vi "INTERFACE.vi"() -> ()   [LabVIEW 2014]
uses:
  <vilib>/regexp/Match Regular Expression.xnode
  <vilib>/Native 3D Graph/xcontrol/3DPC_SurfacePlot.xctl
panel:
  out "Numeric":dbl
  out "Array YZ":cluster{"y":dbl, "z":dbl}[](array[cluster])
  out "Array XZ":cluster{"x":dbl, "z":dbl}[](array[cluster])
  in  "Menu Tab":enum32{"Page 1", "Page 2"}(tab)
  out "IndIOT":bool
  in  "IOT":bool
  out "IndMnC":bool
  in  "Monitoring and\nControlling":bool
  out "IndCon":bool
  in  "Connection":bool
  out "IndMenu":bool
  in  "Menu":bool
  in  "half":bool
  in  "full":bool
  in  "Main Tab":T1(tab)
  in  "POLMAN":bool
  in  "About":bool
  in  "Exit Program":bool
  in  "Help":bool
  in  "Default":bool
  out "connection status":string
  in  "Disconnect Button":bool
  in  "Connect Button":bool
  in  "Port":string
  in  "IP Address":string
  out "Connection Lamp":bool
  in  "Clear Graph 2":bool
  in  "xyzpict":bool
  in  "Tab Mode":enum32{"Manual", "Automatic"}(tab)
  in  "Spindle Speed Default":bool
  in  "Feeed Rate Default":bool
  in  "Back to Home Button 2":bool
  in  "X+ 2":bool
  in  "X- 2":bool
  in  "Y+ 2":bool
  in  "Y- 2":bool
  in  "Z- 2":bool
  in  "Z+ 2":bool
  in  "Back to Origin":bool
  in  "Set Origin":bool
  in  "Length per Step":string(combo)
  out "Dir":string
  in  "Direction":bool
  in  "set spindle speed":bool
  in  "Spindle Speed Knob":dbl(knob) scale=0.0..4000.0
  out "Spindle Speed":dbl
  in  "Feed Rate Knob":dbl(knob) scale=0.0..1000.0
  out "Feed Rate":dbl
  in  "set feed rate":bool
  in  "Spindle OFF":bool
  in  "Spindle ON":bool
  out "Spindle Lamp":bool
  in  "Stop":bool
  in  "Save":bool
  in  "Clear":bool
  in  "Transfer":bool
  in  "Execute":bool
  in  "Insert":bool
  out "File Name":string
  in  "G-Code List":string
  in  "Address":path
  in  "Tab Graphic":enum32{"3D Graph", "PID Graph", "Speed Graph"}(tab)
  in  "Tab Graph":enum32{"XY Graph", "XZ Graph", "YZ Graph"}(tab)
  out "XY Graph":cluster{"X":dbl, "Y":dbl}[](graph)
  out "XZ Graph":cluster{"X":dbl, "Y":dbl}[](graph)
  out "YZ Graph":cluster{"X":dbl, "Y":dbl}[](graph)
  in  "xy":bool
  in  "xz":bool
  in  "yz":bool
  in  "Save PID Button":bool
  in  "Kd":dbl
  in  "Ki":dbl
  in  "Kp":dbl
  out "Waveform Chart":dbl(graph)
  out "Speed Graph":cluster{"X":dbl, "Y":dbl}[](graph)
  in  "Emergency":bool
  out "Green":bool
  out "Yellow":bool
  out "Red":bool
  out "Status":string
  out "X":dbl
  out "Y":dbl
  out "Z":dbl
  in  "Reset":bool
  in  "Clear Graph":bool
  out "Time":dbl
  out "Speed":cluster{"x":dbl, "y":dbl}[](array[cluster])
  out "Array XY":cluster{"x":dbl, "y":dbl}[](array[cluster])
  out "Data Receive":string
  # "C1 2019"
  # "3 D  E N G R A V I N G"
  # "C1 2019"
  # "Teknik Mekatronika\nPoliteknik Manufaktur Bandung"
  # "CONNECT FIRST!"
  # "CONTROL"
  # "INDICATOR"
  # "URGENCY"
  # "SPINDLE"
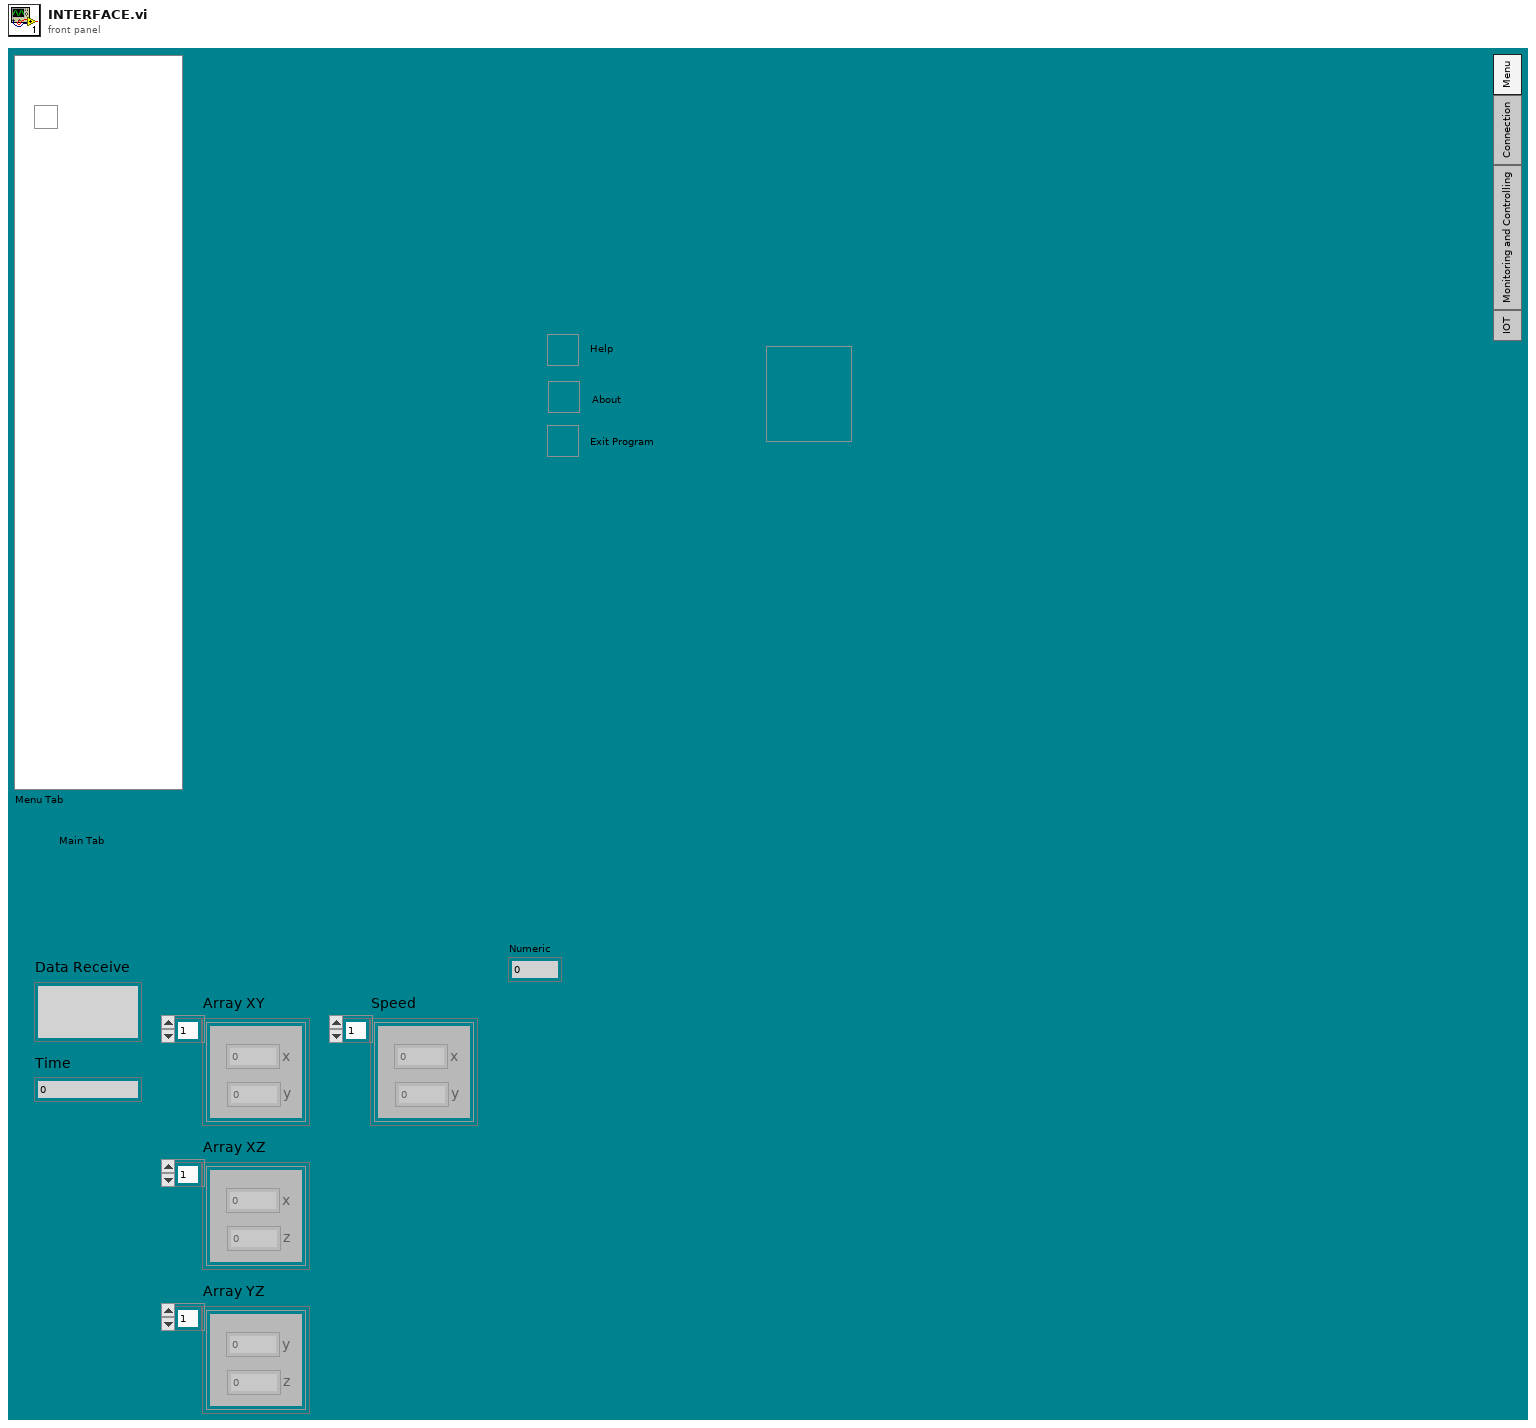
[diagram p1: front panel]
types:
  T1 = enum32{"Menu", "Connection", "Monitoring and Controlling", "IOT"}
  T2 = enum8{"Enabled", "Disabled", "Disabled and Grayed Out"}
  T3 = enum16{"Standard", "Buffered", "CRLF", "Immediate"}
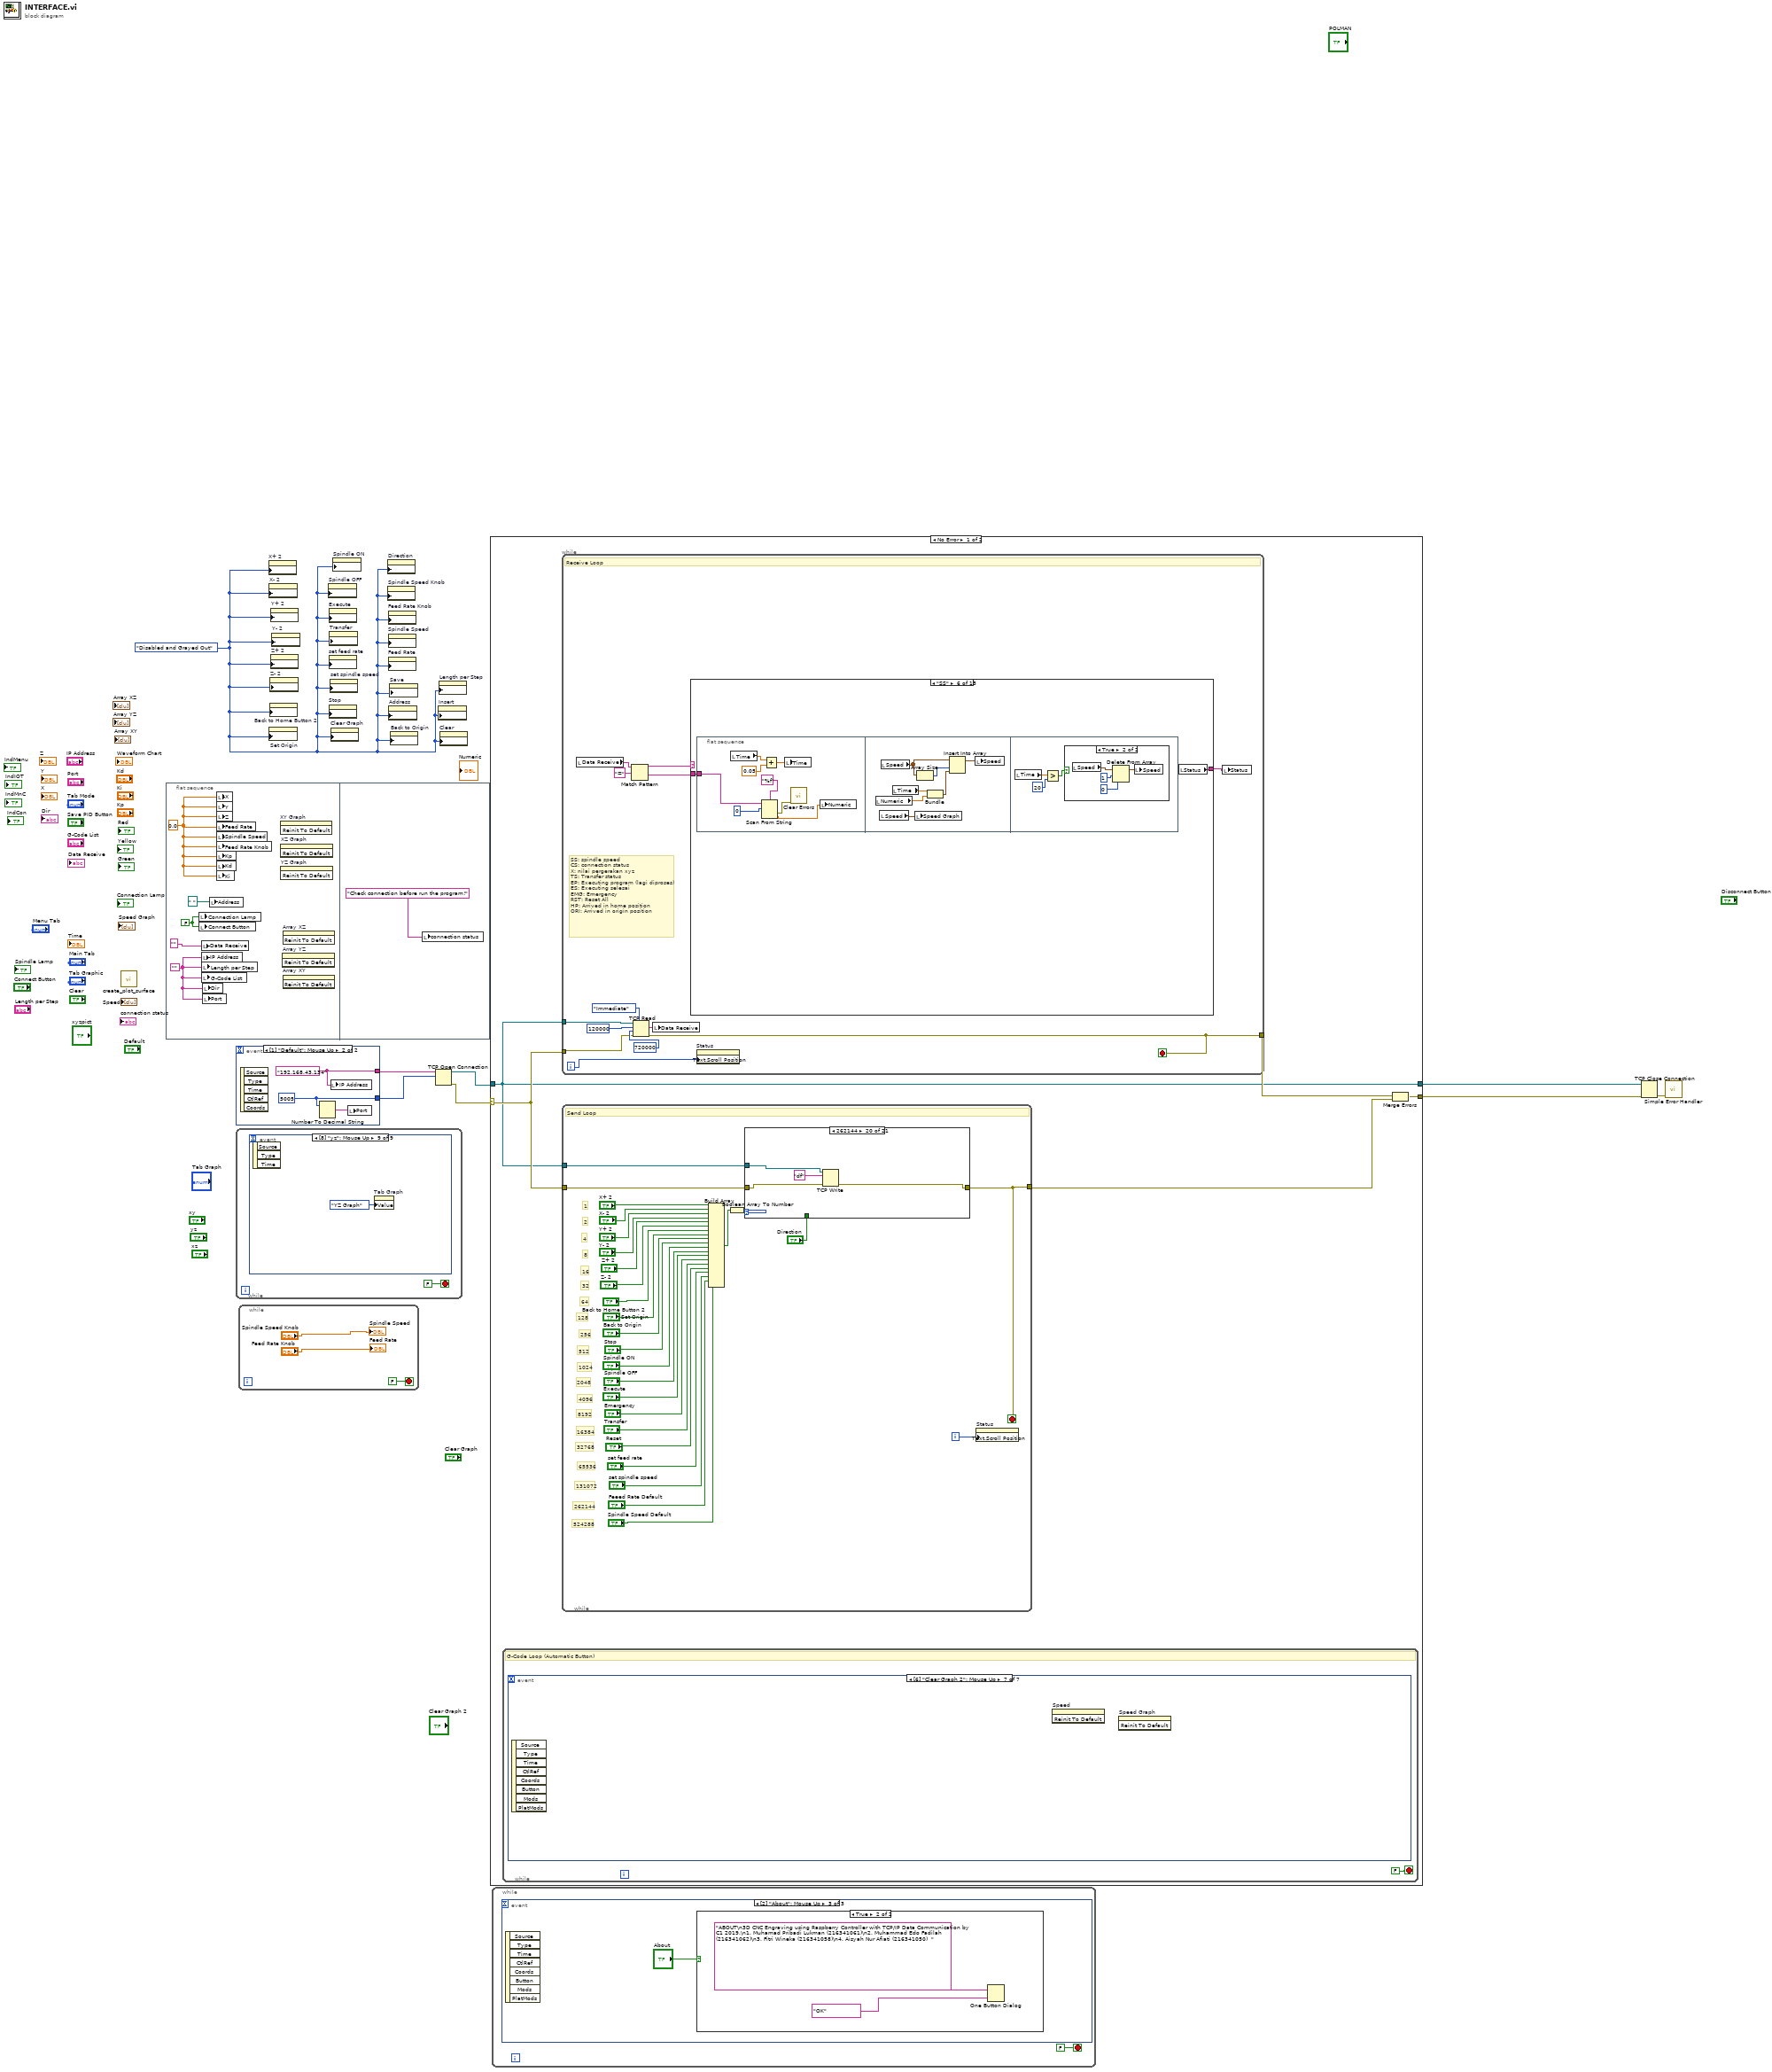
[diagram p0: block diagram]
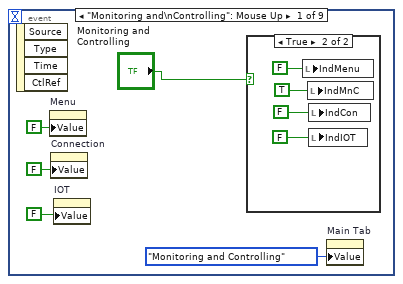
[diagram p2: hidden frame]
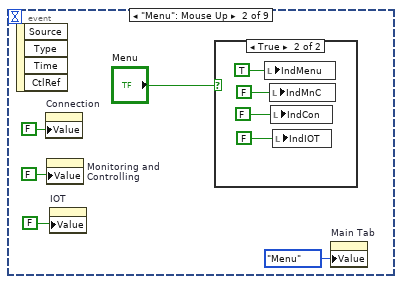
[diagram p4: hidden frame]
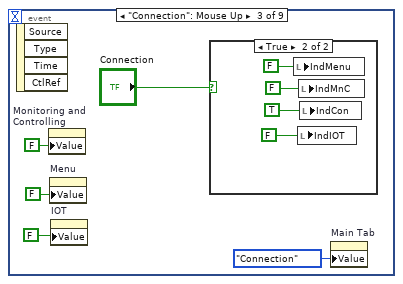
[diagram p6: hidden frame]
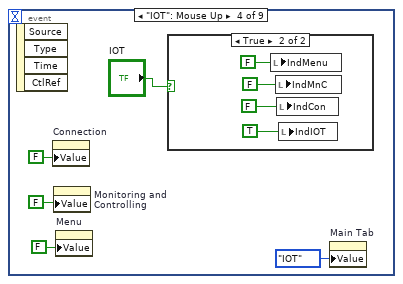
[diagram p8: hidden frame]
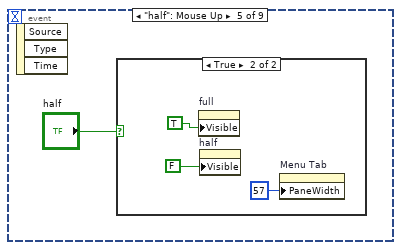
[diagram p10: hidden frame]
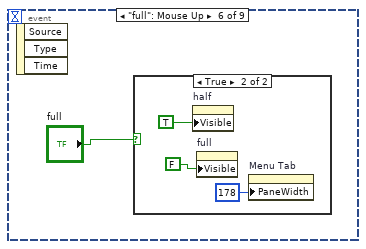
[diagram p12: hidden frame]
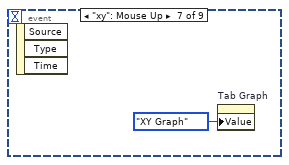
[diagram p14: hidden frame]
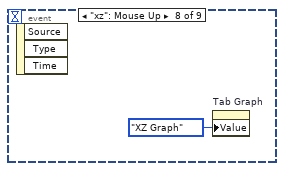
[diagram p15: hidden frame]
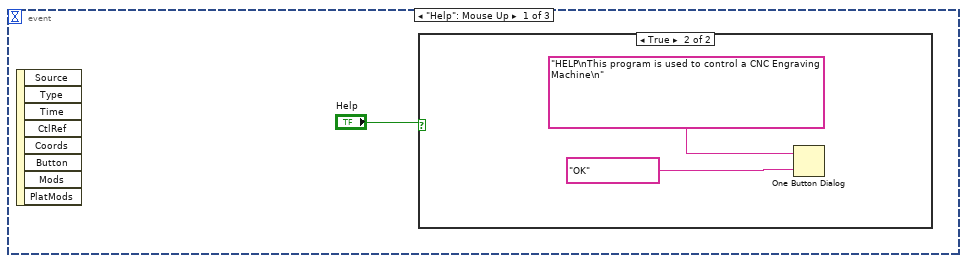
[diagram p16: hidden frame]
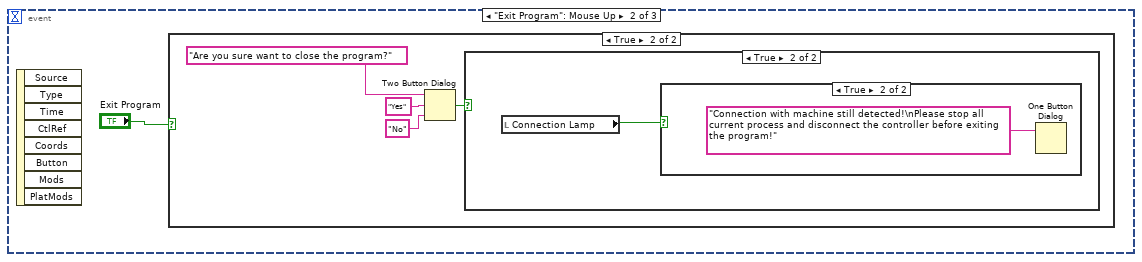
[diagram p18: hidden frame]
diagram:
  w2 = T2."Disabled and Grayed Out" ("Disabled")
  n1 = call <vilib>:"create_plot_surface.vi"() -> ()  [unwired: 5 in, 7 out]
  n2 = flat-sequence {
    frame #0 {
      w11 = FALSE
      w13 = 0.0
      w10 = ""
      n3 = local write "Connection Lamp"(w11) -> ()
      n4 = local write "Connect Button"(w11) -> ()
      n5 = local write "Data Receive"("") -> ()
      n6 = local write "IP Address"(w10) -> ()
      n7 = local write "Length per Step"(w10) -> ()
      n8 = local write "G-Code List"(w10) -> ()
      n9 = local write "Dir"(w10) -> ()
      n10 = local write "Port"(w10) -> ()
      n11 = local write "Address"(path " " ("FILE ADDRESS")) -> ()
      n12 = local write "X"(w13) -> ()
      n13 = local write "Y"(w13) -> ()
      n14 = local write "Z"(w13) -> ()
      n15 = local write "Feed Rate"(w13) -> ()
      n16 = local write "Spindle Speed"(w13) -> ()
      n17 = local write "Feed Rate Knob"(w13) -> ()
      n18 = local write "Kp"(w13) -> ()
      n19 = local write "Kd"(w13) -> ()
      n20 = local write "Ki"(w13) -> ()
      n21 = invoke on="XY Graph" class="XYGraph (strict)" method="Reinit To Default"() -> ()  [unwired: 3 in, 3 out]
      n22 = invoke on="XZ Graph" class="XYGraph (strict)" method="Reinit To Default"() -> ()  [unwired: 3 in, 3 out]
      n23 = invoke on="YZ Graph" class="XYGraph (strict)" method="Reinit To Default"() -> ()  [unwired: 3 in, 3 out]
      n24 = invoke on="Array YZ" class="Arr (strict)" method="Reinit To Default"() -> ()  [unwired: 3 in, 3 out]
      n25 = invoke on="Array XZ" class="Arr (strict)" method="Reinit To Default"() -> ()  [unwired: 3 in, 3 out]
      n26 = invoke on="Array XY" class="Arr (strict)" method="Reinit To Default"() -> ()  [unwired: 3 in, 3 out]
    }
    frame #1 {
      n27 = local write "connection status"("Check connection before run the program!" ("STATUS")) -> ()
    }
  }
  n28 = event shown="[1] \"Default\": Mouse Up" {
    selector: _ -> [_ _]
    dyn-events: _ -> [_ _]
    timeout: _ -> [_ _]
    tunnel: [w17 w20] -> w3
    tunnel: [w15 w18] -> w1
    event "Connect Button": Value Change {
      n29 = event-data() -> ()  [unwired: 1 in, 5 out]
      n30 = local read "Port"() -> (w16:string)
      n31 = local read "IP Address"() -> (w17:string)
      n32 = Decimal String To Number(string=w16) -> (number=w15:i32)  [unwired: 2 in, 1 out]
    }
    event "Default": Mouse Up {
      w20 = "192.168.43.134"
      w18 = 5005
      n33 = event-data() -> ()  [unwired: 1 in, 5 out]
      n34 = Number To Decimal String(number=w18) -> (decimal integer string=w19:string)  [unwired: 1 in]
      n35 = local write "IP Address"(w20) -> ()
      n36 = local write "Port"(w19) -> ()
    }
  }
  n37 = while {
    stop <- FALSE stop-if-true
    n38 = event shown="[8] \"yz\": Mouse Up" {
      selector: _ -> [_ _ _ _ _ _ _ _ _]
      dyn-events: _ -> [_ _ _ _ _ _ _ _ _]
      timeout: _ -> [_ _ _ _ _ _ _ _ _]
      event "Monitoring and\nControlling": Mouse Up {
        n39 = event-data() -> ()  [unwired: 1 in, 4 out]
        n40 = property on="Menu" class="Bool (strict)"("Value"=FALSE ("Menu")) -> ()  [unwired: 2 in, 2 out]
        n41 = property on="Connection" class="Bool (strict)"("Value"=FALSE ("Connection")) -> ()  [unwired: 2 in, 2 out]
        n42 = property on="IOT" class="Bool (strict)"("Value"=FALSE ("Connection")) -> ()  [unwired: 2 in, 2 out]
        n43 = case shown="True" "Monitoring and\nControlling" {
          frame False {
          }
          frame True {
            n44 = local write "IndMenu"(FALSE) -> ()
            n45 = local write "IndMnC"(TRUE) -> ()
            n46 = local write "IndCon"(FALSE) -> ()
            n47 = local write "IndIOT"(FALSE) -> ()
          }
        }
        n48 = property on="Main Tab" class="TabCtl (strict)"("Value"=T1."Monitoring and Controlling" ("Main Tab")) -> ()  [unwired: 2 in, 2 out]
      }
      event "Menu": Mouse Up {
        n49 = event-data() -> ()  [unwired: 1 in, 4 out]
        n50 = property on="Connection" class="Bool (strict)"("Value"=FALSE ("Connection")) -> ()  [unwired: 2 in, 2 out]
        n51 = property on="Monitoring and\nControlling" class="Bool (strict)"("Value"=FALSE ("Connection")) -> ()  [unwired: 2 in, 2 out]
        n52 = property on="IOT" class="Bool (strict)"("Value"=FALSE ("Connection")) -> ()  [unwired: 2 in, 2 out]
        n53 = case shown="True" "Menu" {
          frame False {
          }
          frame True {
            n54 = local write "IndMenu"(TRUE) -> ()
            n55 = local write "IndMnC"(FALSE) -> ()
            n56 = local write "IndCon"(FALSE) -> ()
            n57 = local write "IndIOT"(FALSE) -> ()
          }
        }
        n58 = property on="Main Tab" class="TabCtl (strict)"("Value"=T1."Menu" ("Main Tab")) -> ()  [unwired: 2 in, 2 out]
      }
      event "Connection": Mouse Up {
        n59 = event-data() -> ()  [unwired: 1 in, 4 out]
        n60 = property on="Monitoring and\nControlling" class="Bool (strict)"("Value"=FALSE ("Monitoring and Controlling")) -> ()  [unwired: 2 in, 2 out]
        n61 = property on="Menu" class="Bool (strict)"("Value"=FALSE ("Menu")) -> ()  [unwired: 2 in, 2 out]
        n62 = property on="IOT" class="Bool (strict)"("Value"=FALSE ("Connection")) -> ()  [unwired: 2 in, 2 out]
        n63 = case shown="True" "Connection" {
          frame False {
          }
          frame True {
            n64 = local write "IndMenu"(FALSE) -> ()
            n65 = local write "IndIOT"(FALSE) -> ()
            n66 = local write "IndMnC"(FALSE) -> ()
            n67 = local write "IndCon"(TRUE) -> ()
          }
        }
        n68 = property on="Main Tab" class="TabCtl (strict)"("Value"=T1."Connection" ("Main Tab")) -> ()  [unwired: 2 in, 2 out]
      }
      event "IOT": Mouse Up {
        n69 = event-data() -> ()  [unwired: 1 in, 4 out]
        n70 = property on="Connection" class="Bool (strict)"("Value"=FALSE ("Connection")) -> ()  [unwired: 2 in, 2 out]
        n71 = property on="Monitoring and\nControlling" class="Bool (strict)"("Value"=FALSE ("Connection")) -> ()  [unwired: 2 in, 2 out]
        n72 = property on="Menu" class="Bool (strict)"("Value"=FALSE ("Menu")) -> ()  [unwired: 2 in, 2 out]
        n73 = case shown="True" "IOT" {
          frame False {
          }
          frame True {
            n74 = local write "IndMenu"(FALSE) -> ()
            n75 = local write "IndMnC"(FALSE) -> ()
            n76 = local write "IndCon"(FALSE) -> ()
            n77 = local write "IndIOT"(TRUE) -> ()
          }
        }
        n78 = property on="Main Tab" class="TabCtl (strict)"("Value"=T1."IOT" ("Main Tab")) -> ()  [unwired: 2 in, 2 out]
      }
      event "half": Mouse Up {
        n79 = event-data() -> ()  [unwired: 1 in, 3 out]
        n80 = case shown="True" "half" {
          frame False {
          }
          frame True {
            n81 = property on="full" class="Bool (strict)"("Visible"=TRUE) -> ()  [unwired: 2 in, 2 out]
            n82 = property on="half" class="Bool (strict)"("Visible"=FALSE) -> ()  [unwired: 2 in, 2 out]
            n83 = property on="Menu Tab" class="TabCtl (strict)"("PaneWidth"=u32 57 ("Tab Control Pane Dimension:Height")) -> ()  [unwired: 2 in, 2 out]
          }
        }
      }
      event "full": Mouse Up {
        n84 = event-data() -> ()  [unwired: 1 in, 3 out]
        n85 = case shown="True" "full" {
          frame False {
          }
          frame True {
            n86 = property on="half" class="Bool (strict)"("Visible"=TRUE) -> ()  [unwired: 2 in, 2 out]
            n87 = property on="full" class="Bool (strict)"("Visible"=FALSE) -> ()  [unwired: 2 in, 2 out]
            n88 = property on="Menu Tab" class="TabCtl (strict)"("PaneWidth"=u32 178 ("Tab Control Pane Dimension:Height")) -> ()  [unwired: 2 in, 2 out]
          }
        }
      }
      event "xy": Mouse Up {
        n89 = event-data() -> ()  [unwired: 1 in, 3 out]
        n90 = property on="Tab Graph" class="TabCtl (strict)"("Value"=enum32{"XY Graph", "XZ Graph", "YZ Graph"}."XY Graph" ("Tab Graph")) -> ()  [unwired: 2 in, 2 out]
      }
      event "xz": Mouse Up {
        n91 = event-data() -> ()  [unwired: 1 in, 3 out]
        n92 = property on="Tab Graph" class="TabCtl (strict)"("Value"=enum32{"XY Graph", "XZ Graph", "YZ Graph"}."XZ Graph" ("Tab Graph")) -> ()  [unwired: 2 in, 2 out]
      }
      event "yz": Mouse Up {
        n93 = event-data() -> ()  [unwired: 1 in, 3 out]
        n94 = property on="Tab Graph" class="TabCtl (strict)"("Value"=enum32{"XY Graph", "XZ Graph", "YZ Graph"}."YZ Graph" ("Tab Graph")) -> ()  [unwired: 2 in, 2 out]
      }
    }
  }
  n95 = while {
    stop <- FALSE stop-if-true
    "Feed Rate" <- "Feed Rate Knob"
    "Spindle Speed" <- "Spindle Speed Knob"
  }
  n96 = property on="X+ 2" class="Bool"("DisabledEnum"=w2) -> ()  [unwired: 2 in, 2 out]
  n97 = property on="X- 2" class="Bool"("DisabledEnum"=w2) -> ()  [unwired: 2 in, 2 out]
  n98 = property on="Set Origin" class="Bool"("DisabledEnum"=w2) -> ()  [unwired: 2 in, 2 out]
  n99 = property on="Back to Home Button 2" class="Bool"("DisabledEnum"=w2) -> ()  [unwired: 2 in, 2 out]
  n100 = property on="Z- 2" class="Bool"("DisabledEnum"=w2) -> ()  [unwired: 2 in, 2 out]
  n101 = property on="Y+ 2" class="Bool"("DisabledEnum"=w2) -> ()  [unwired: 2 in, 2 out]
  n102 = property on="Z+ 2" class="Bool"("DisabledEnum"=w2) -> ()  [unwired: 2 in, 2 out]
  n103 = property on="Y- 2" class="Bool"("DisabledEnum"=w2) -> ()  [unwired: 2 in, 2 out]
  n104 = property on="Spindle OFF" class="Bool"("DisabledEnum"=w2) -> ()  [unwired: 2 in, 2 out]
  n105 = property on="Execute" class="Bool"("DisabledEnum"=w2) -> ()  [unwired: 2 in, 2 out]
  n106 = property on="set feed rate" class="Bool"("DisabledEnum"=w2) -> ()  [unwired: 2 in, 2 out]
  n107 = property on="Stop" class="Bool"("DisabledEnum"=w2) -> ()  [unwired: 2 in, 2 out]
  n108 = property on="Transfer" class="Bool"("DisabledEnum"=w2) -> ()  [unwired: 2 in, 2 out]
  n109 = property on="set spindle speed" class="Bool"("DisabledEnum"=w2) -> ()  [unwired: 2 in, 2 out]
  n110 = property on="Clear Graph" class="Bool (strict)"("DisabledEnum"=w2) -> ()  [unwired: 2 in, 2 out]
  n111 = property on="Spindle ON" class="Bool"("DisabledEnum"=w2) -> ()  [unwired: 2 in, 2 out]
  n112 = property on="Direction" class="Bool (strict)"("DisabledEnum"=w2) -> ()  [unwired: 2 in, 2 out]
  n113 = property on="Spindle Speed Knob" class="Knob (strict)"("DisabledEnum"=w2) -> ()  [unwired: 2 in, 2 out]
  n114 = property on="Feed Rate Knob" class="Knob (strict)"("DisabledEnum"=w2) -> ()  [unwired: 2 in, 2 out]
  n115 = property on="Spindle Speed" class="DigNum (strict)"("DisabledEnum"=w2) -> ()  [unwired: 2 in, 2 out]
  n116 = property on="Feed Rate" class="DigNum (strict)"("DisabledEnum"=w2) -> ()  [unwired: 2 in, 2 out]
  n117 = property on="Address" class="Path"("DisabledEnum"=w2) -> ()  [unwired: 2 in, 2 out]
  n118 = property on="Save" class="Bool (strict)"("DisabledEnum"=w2) -> ()  [unwired: 2 in, 2 out]
  n119 = property on="Back to Origin" class="Bool"("DisabledEnum"=w2) -> ()  [unwired: 2 in, 2 out]
  n120 = TCP Open Connection(address=w3, remote port or service name=w1) -> (connection ID=w7:refnum<k5>, error out=w8:errorcluster)  [unwired: 3 in]
  n121 = property on="Insert" class="Bool (strict)"("DisabledEnum"=w2) -> ()  [unwired: 2 in, 2 out]
  n122 = property on="Length per Step" class="CmbBox"("DisabledEnum"=w2) -> ()  [unwired: 2 in, 2 out]
  n123 = property on="Clear" class="Bool (strict)"("DisabledEnum"=w2) -> ()  [unwired: 2 in, 2 out]
  n124 = case shown="No Error" w8 {
    selector: w8 -> [w75 w1079]
    tunnel: w7 -> [w74 w1080]
    tunnel: [w72 w1079] -> w6
    tunnel: [w74 w1080] -> w4
    frame No Error {
      n125 = while {
        stop <- FALSE stop-if-true
        # "G-Code Loop (Automatic Button)"
        n126 = event shown="[6] \"Clear Graph 2\": Mouse Up" {
          selector: _ -> [_ _ _ _ _ _ _]
          dyn-events: _ -> [_ _ _ _ _ _ _]
          timeout: _ -> [_ _ _ _ _ _ _]
          event "Insert": Mouse Up {
            n127 = event-data() -> ()  [unwired: 1 in, 8 out]
            n128 = case shown="True" "Insert" {
              frame False {
              }
              frame True {
                w84 = "Open G-Code Manually"  # prompt (open existing file)
                n129 = Read from Text File(prompt (Open existing file)=w84) -> (refnum out=w80:refnum<file>, text=w82:string, cancelled=w81:bool, error out=w83:errorcluster)  [unwired: 3 in]
                n130 = call <vilib>:"Clear Errors.vi"("error in (no error)"=w83) -> ()  [unwired: 5 in, 2 out]
                n131 = case shown="False" w81 {
                  tunnel: w82 -> [_ w90]
                  tunnel: ["Cancelled" w89] -> w79
                  tunnel: w80 -> [_ w87]
                  frame True {
                  }
                  frame False {
                    n132 = Refnum to Path(1:w87) -> (0:w95:path)
                    n133 = Strip Path(path=w95) -> (name=w91:string)  [unwired: 1 out]
                    n134 = xnode ("Match Regular Expression")("input string"=w91, "regular expression"=".nc", "ignore case? (F)"=TRUE) -> ("whole match"=w94:string)  [unwired: 3 in, 4 out]
                    n135 = Printable?(1:w94) -> (0:w88:bool)
                    n136 = case shown="False" w88 {
                      tunnel: ["File is not compatible." "File opened"] -> w89
                      tunnel: w91 -> [_ _]
                      tunnel: w90 -> [_ w100]
                      tunnel: ["" w100] -> w86
                      frame False {
                        n137 = One Button Dialog(message="The file you are trying to open is not compatible with this program.", button name ("OK")="OK") -> ()  [unwired: 1 out]
                      }
                      frame True {
                      }
                    }
                    n138 = local write "G-Code List"(w86) -> ()
                  }
                }
                n139 = local write "Status"(w79) -> ()
              }
            }
          }
          event "Address": Value Change {
            n140 = event-data() -> ()  [unwired: 1 in, 6 out]
            n141 = flat-sequence {
              tunnel: [w224] -> w219
              tunnel: [w223] -> w218
              tunnel: [w222] -> w217
              tunnel: [w221] -> w216
              tunnel: w219 -> [w493]
              tunnel: w218 -> [w494]
              tunnel: w217 -> [w495]
              tunnel: w216 -> [w496]
              frame #0 {
                n142 = Strip Path(path="Address") -> (stripped path=w236:path, name=w235:string)
                n143 = xnode "Match Regular Expression"("input string"=w235, "regular expression"=".dxf", "ignore case? (F)"=FALSE) -> ("before match"=w233:string, "whole match"=w232:string)  [unwired: 3 in, 3 out]
                n144 = Printable?(1:w232) -> (0:w225:bool)
                n145 = case shown="False" w225 {
                  tunnel: w236 -> [w372 w488]
                  tunnel: w235 -> [w369 w489]
                  tunnel: w233 -> [_ w490]
                  tunnel: "Address" -> [w365 w487]
                  tunnel: [w366 FALSE] -> w226
                  tunnel: [w367 w490] -> w227
                  tunnel: [w369 w489] -> w229
                  tunnel: [w372 w488] -> w228
                  tunnel: [w365 w487] -> w230
                  frame False {
                    n146 = xnode "Match Regular Expression"("input string"=w369, "regular expression"=".stl", "ignore case? (F)"=TRUE) -> ("before match"=w367:string, "whole match"=w368:string)  [unwired: 3 in, 3 out]
                    n147 = Printable?(1:w368) -> (0:w366:bool)
                  }
                  frame True {
                  }
                }
                n148 = Or(x=w226, y=w225) -> (x .or. y?=w221:bool)
                n149 = case shown="False" w221 {
                  tunnel: w230 -> [_ w250]
                  tunnel: w229 -> [_ w243]
                  tunnel: w228 -> [_ w242]
                  tunnel: w227 -> [_ w241]
                  tunnel: [w238 w243] -> w223
                  tunnel: [w237 w242] -> w224
                  tunnel: [w238 w241] -> w222
                  frame False {
                    w238 = ""
                    w237 = path ""
                    n150 = One Button Dialog(message="The file you are trying to open is not compatible with this program.", button name ("OK")="OK") -> ()  [unwired: 1 out]
                    n151 = local write "Address"(w237) -> ()
                  }
                  frame True {
                    n152 = Path To String(path=w250) -> (string=w248:string)
                    n153 = Concatenate Strings("cmd /c\"", w248, "\"") -> (w246:string)
                    n154 = call <vilib>:"System Exec.vi"("run minimized? (F)"=FALSE, "wait until completion? (T)"=TRUE, "command line"=w246) -> ()  [unwired: 5 in, 4 out]
                  }
                }
              }
              frame #1 {
                n155 = case shown="True" w496 {
                  tunnel: w495 -> [_ w506]
                  tunnel: w494 -> [_ w498]
                  tunnel: w493 -> [_ w503]
                  tunnel: ["File is not compatible." w499] -> w492
                  frame False {
                  }
                  frame True {
                    n156 = Concatenate Strings(w506, ".nc") -> (w504:string)
                    n157 = Build Path(base path=w503, name or relative path=w504) -> (appended path=w502:path)
                    n158 = Read from Text File(file (use dialog)=w502) -> (text=w500:string, error out=w501:errorcluster)  [unwired: 3 in, 2 out]
                    n159 = case shown="Error" w501 {
                      tunnel: w500 -> [_ _]
                      tunnel: ["File opened" w508] -> w499
                      frame No Error {
                      }
                      frame Error {
                        n160 = Two Button Dialog(message="Your G-Code file may has different name or location as your 3D file. Do you want to browse it manually?", 1:"No", 2:"Yes") -> (T button?=w509:bool)
                        n161 = case shown="True" w509 {
                          tunnel: ["Cancelled" w514] -> w508
                          frame False {
                          }
                          frame True {
                            n162 = Read from Text File(prompt (Open existing file)="Open G-Code manually") -> (refnum out=w515:refnum<file>, text=w516:string, cancelled=w517:bool, error out=w518:errorcluster)  [unwired: 3 in]
                            n163 = call <vilib>:"Clear Errors.vi"("error in (no error)"=w518) -> ()  [unwired: 5 in, 2 out]
                            n164 = case shown="False" w517 {
                              tunnel: w516 -> [w525 _]
                              tunnel: w515 -> [w531 _]
                              tunnel: [w522 "Cancelled"] -> w514
                              frame False {
                                n165 = Refnum to Path(1:w531) -> (0:w524:path)
                                n166 = Strip Path(path=w524) -> (name=w526:string)  [unwired: 1 out]
                                n167 = xnode "Match Regular Expression"("input string"=w526, "regular expression"=".nc", "ignore case? (F)"=TRUE) -> ("whole match"=w528:string)  [unwired: 3 in, 4 out]
                                n168 = Printable?(1:w528) -> (0:w527:bool)
                                n169 = case shown="False" w527 {
                                tunnel: w526 -> [_ w539]
                                tunnel: w525 -> [_ w538]
                                tunnel: w524 -> [_ w540]
                                tunnel: [path "" w540] -> w521
                                tunnel: [w534 w539] -> w523
                                tunnel: [w534 w538] -> w520
                                tunnel: ["File is not compatible" "File opened"] -> w522
                                frame False {
                                w534 = ""
                                n170 = One Button Dialog(message="The file you are trying to open has different file format.", button name ("OK")="OK") -> ()  [unwired: 1 out]
                                }
                                frame True {
                                }
                                }
                                n171 = local write "File Name"(w523) -> ()
                                n172 = local write "G-Code List"(w520) -> ()
                                n173 = local write "Address"(w521) -> ()
                              }
                              frame True {
                              }
                            }
                          }
                        }
                      }
                    }
                    "File Name" <- w498
                  }
                }
                "Status" <- w492
              }
            }
          }
          event "Save": Value Change {
            n174 = event-data() -> ()  [unwired: 1 in, 6 out]
            n175 = case shown="True" "Save" {
              frame False {
              }
              frame True {
                n176 = property on="G-Code List" class="Str"() -> ("Text.Text"=w657:string)  [unwired: 2 in, 2 out]
                n177 = Write to Text File(prompt (Choose or enter file path)="Save", text=w657) -> (cancelled=w660:bool, error out=w659:errorcluster)  [unwired: 2 in, 1 out]
                n178 = case shown="True" w660 {
                  tunnel: ["G-Code file is saved" "Cancelled saving"] -> w658
                  frame False {
                  }
                  frame True {
                  }
                }
                n179 = call <vilib>:"Clear Errors.vi"("error in (no error)"=w659) -> ()  [unwired: 5 in, 2 out]
                n180 = local write "Status"(w658) -> ()
              }
            }
          }
          event "Reset": Mouse Up {
            w664 = ""
            n181 = event-data() -> ()  [unwired: 1 in, 8 out]
            n182 = local write "File Name"(w664) -> ()
            n183 = local write "Address"(path "") -> ()
            n184 = local write "G-Code List"(w664) -> ()
            n185 = local write "Status"(w664) -> ()
          }
          event "Clear": Mouse Up {
            w667 = ""
            n186 = event-data() -> ()  [unwired: 1 in, 8 out]
            n187 = local write "Length per Step"(w667) -> ()
            n188 = local write "G-Code List"(w667) -> ()
            n189 = local write "File Name"(w667) -> ()
            n190 = local write "Status"(w667) -> ()
            n191 = local write "Address"(path "") -> ()
          }
          event "Clear Graph": Mouse Up {
            w668 = 0.0
            n192 = event-data() -> ()  [unwired: 1 in, 8 out]
            n193 = invoke on="XY Graph" class="XYGraph (strict)" method="Reinit To Default"() -> ()  [unwired: 3 in, 3 out]
            n194 = invoke on="XZ Graph" class="XYGraph (strict)" method="Reinit To Default"() -> ()  [unwired: 3 in, 3 out]
            n195 = invoke on="YZ Graph" class="XYGraph (strict)" method="Reinit To Default"() -> ()  [unwired: 3 in, 3 out]
            n196 = invoke on="Array YZ" class="Arr (strict)" method="Reinit To Default"() -> ()  [unwired: 3 in, 3 out]
            n197 = invoke on="Array XZ" class="Arr (strict)" method="Reinit To Default"() -> ()  [unwired: 3 in, 3 out]
            n198 = invoke on="Array XY" class="Arr (strict)" method="Reinit To Default"() -> ()  [unwired: 3 in, 3 out]
            n199 = local write "X"(w668) -> ()
            n200 = local write "Y"(w668) -> ()
            n201 = local write "Z"(w668) -> ()
          }
          event "Clear Graph 2": Mouse Up {
            n202 = event-data() -> ()  [unwired: 1 in, 8 out]
            n203 = invoke on="Speed" class="Arr (strict)" method="Reinit To Default"() -> ()  [unwired: 3 in, 3 out]
            n204 = invoke on="Speed Graph" class="XYGraph (strict)" method="Reinit To Default"() -> ()  [unwired: 3 in, 3 out]
          }
        }
      }
      n205 = while {
        tunnel: w74 -> [w901]
        tunnel: w75 -> [w900]
        tunnel: [w899] -> w76
        i -> [w898]
        stop <- w899 stop-if-true
        # "SS: spindle speed\nCS: connection status\nX: nilai pergerakan xyz\nTS: Transfer status\nEP: Executing program (lagi diproses)\nES: Executing selesai\nEMG: Emergency\nRST: Reset All\nHP: Arrived in home position\nORI: Arrived in origin position"
        # "Receive Loop"
        n206 = local read "Data Receive"() -> (w895:string)
        n207 = Match Pattern(string=w895, regular expression="=") -> (before substring=w897:string, after substring=w893:string)  [unwired: 1 in, 2 out]
        n208 = TCP Read(connection ID=w901, bytes to read=120000, error in (no error)=w900, 7:T3."Immediate" ("mode (standard)"), 9:720000) -> (data out=w902:string, error out=w899:errorcluster)  [unwired: 1 out]
        n209 = local write "Data Receive"(w902) -> ()
        n210 = case shown="\"SS\"" w897 {
          tunnel: w893 -> [_ w907 _ _ _ w976 _ _ _ _ _ _ _]
          tunnel: [w906 w908 w943 w956 w966 w977 "" w1008 w1026 w1036 w1046 w1057 w1067] -> w894
          frame "0", Default {
            n211 = local read "Status"() -> (w906:string)
          }
          frame "X" {
            n212 = flat-sequence {
              tunnel: w907 -> [w909]
              frame #0 {
                n213 = Scan From String "Scan From String"(format string="%fY%fZ%f", input string=w909, initial scan location=u32 0) -> (error out=w914:errorcluster, output 1=w912:dbl, output 2=w911:dbl, output 3=w910:dbl)  [unwired: 4 in, 2 out]
                n214 = call <vilib>:"Clear Errors.vi"("error in (no error)"=w914) -> ()  [unwired: 5 in, 2 out]
                n215 = local write "X"(w912) -> ()
                n216 = local write "Y"(w911) -> ()
                n217 = local write "Z"(w910) -> ()
              }
              frame #1 {
                n218 = local read "Array XY"() -> (w941:cluster{"x":dbl, "y":dbl}[])
                n219 = local read "X"() -> (w925:dbl)
                n220 = local read "Y"() -> (w926:dbl)
                n221 = local read "Array XZ"() -> (w936:cluster{"x":dbl, "z":dbl}[])
                n222 = local read "X"() -> (w923:dbl)
                n223 = local read "Z"() -> (w924:dbl)
                n224 = local read "Array YZ"() -> (w935:cluster{"y":dbl, "z":dbl}[])
                n225 = local read "Y"() -> (w922:dbl)
                n226 = local read "Z"() -> (w933:dbl)
                n227 = local read "Array XY"() -> (w918:cluster{"x":dbl, "y":dbl}[])
                n228 = local read "Array XZ"() -> (w917:cluster{"x":dbl, "z":dbl}[])
                n229 = local read "Array YZ"() -> (w916:cluster{"y":dbl, "z":dbl}[])
                n230 = Array Size(array=w941) -> (size(s)=w939:i32)
                n231 = Bundle("X"=w925, "Y"=w926) -> (w940:cluster{"X":dbl, "Y":dbl})  [unwired: 1 in]
                n232 = Bundle("Y"=w926, "X"=w925) -> (w921:cluster{"Y":dbl, "X":dbl})  [unwired: 1 in]
                n233 = Array Size(array=w936) -> (size(s)=w938:i32)
                n234 = Bundle("X"=w923, "Z"=w924) -> (w937:cluster{"X":dbl, "Z":dbl})  [unwired: 1 in]
                n235 = Bundle("Z"=w924, "X"=w923) -> (w920:cluster{"Z":dbl, "X":dbl})  [unwired: 1 in]
                n236 = Array Size(array=w935) -> (size(s)=w932:i32)
                n237 = Bundle("Y"=w922, "Z"=w933) -> (w934:cluster{"Y":dbl, "Z":dbl})  [unwired: 1 in]
                n238 = Bundle("Y"=w922, "Y"=w922) -> (w919:cluster{"Y":dbl, "Y":dbl})  [unwired: 1 in]
                n239 = Insert Into Array(array=w941, index=w939, new element=w940) -> (w942:cluster{"x":dbl, "y":dbl}[])
                n240 = Insert Into Array(array=w936, index=w938, new element=w937) -> (w931:cluster{"x":dbl, "z":dbl}[])
                n241 = Build Array (concatenate)(w921, w918) -> (→"XY Graph":cluster{"x":dbl, "y":dbl}[])
                n242 = Build Array (concatenate)(w920, w917) -> (→"XZ Graph":cluster{"x":dbl, "z":dbl}[])
                n243 = Insert Into Array(array=w935, index=w932, new element=w934) -> (w930:cluster{"y":dbl, "z":dbl}[])
                n244 = Build Array (concatenate)(w919, w916) -> (→"YZ Graph":cluster{"y":dbl, "z":dbl}[])
                n245 = local write "Array XY"(w942) -> ()
                n246 = local write "Array YZ"(w930) -> ()
                n247 = local write "Array XZ"(w931) -> ()
              }
            }
            n248 = local read "Status"() -> (w908:string)
          }
          frame "TS" {
            n249 = local read "Status"() -> (w947:string)
            n250 = Equal?(x=w947, y="") -> (x = y?=w945:bool)
            n251 = case shown="False" w945 {
              tunnel: "G-Code is transferred successfully.\nYou may execute the program" -> [w948 w952]
              tunnel: [w949 w952] -> w943
              frame False {
                n252 = local read "Status"() -> (w950:string)
                n253 = Concatenate Strings(w950, "\r", w948) -> (w949:string)
              }
              frame True {
              }
            }
          }
          frame "EP" {
            n254 = local read "Status"() -> (w957:string)
            n255 = local write "Yellow"(FALSE) -> ()
            n256 = local write "Green"(TRUE) -> ()
            n257 = local write "Red"(FALSE) -> ()
            n258 = Equal?(x=w957, y="") -> (x = y?=w959:bool)
            n259 = case shown="False" w959 {
              tunnel: "Executing the program..." -> [w962 w965]
              tunnel: [w961 w965] -> w956
              frame False {
                n260 = local read "Status"() -> (w963:string)
                n261 = Concatenate Strings(w963, "\r", w962) -> (w961:string)
              }
              frame True {
              }
            }
          }
          frame "ES" {
            n262 = local read "Status"() -> (w968:string)
            n263 = Equal?(x=w968, y="") -> (x = y?=w967:bool)
            n264 = case shown="False" w967 {
              tunnel: "The program has been fully executed" -> [w972 w975]
              tunnel: [w971 w975] -> w966
              frame False {
                n265 = local read "Status"() -> (w974:string)
                n266 = Concatenate Strings(w974, "\r", w972) -> (w971:string)
              }
              frame True {
              }
            }
          }
          frame "SS" {
            n267 = flat-sequence {
              tunnel: w976 -> [w982]
              frame #0 {
                n268 = local read "Time"() -> (w985:dbl)
                n269 = Scan From String "Scan From String"(format string="%f", input string=w982, initial scan location=u32 0) -> (error out=w981:errorcluster, output 1=w978:dbl)  [unwired: 2 in, 2 out]
                n270 = Add(x=w985, y=0.05) -> (x+y=w983:dbl)
                n271 = local write "Time"(w983) -> ()
                n272 = call <vilib>:"Clear Errors.vi"("error in (no error)"=w981) -> ()  [unwired: 5 in, 2 out]
                n273 = local write "Numeric"(w978) -> ()
              }
              frame #1 {
                n274 = local read "Numeric"() -> (w989:dbl)
                n275 = local read "Speed"() -> (w986:cluster{"x":dbl, "y":dbl}[])
                n276 = local read "Speed"() -> (w991:cluster{"x":dbl, "y":dbl}[])
                n277 = local read "Time"() -> (w988:dbl)
                n278 = local write "Speed Graph"(w986) -> ()
                n279 = Array Size(array=w991) -> (size(s)=w992:i32)
                n280 = Bundle("Time"=w988, "Numeric"=w989) -> (w987:cluster{"Time":dbl, "Numeric":dbl})  [unwired: 1 in]
                n281 = Insert Into Array(array=w991, index=w992, new element=w987) -> (w990:cluster{"x":dbl, "y":dbl}[])
                n282 = local write "Speed"(w990) -> ()
              }
              frame #2 {
                n283 = local read "Time"() -> (w995:dbl)
                n284 = Greater?(x=w995, y=20) -> (0:w994:bool)
                n285 = case shown="True" w994 {
                  frame False {
                  }
                  frame True {
                    n286 = local read "Speed"() -> (w997:cluster{"x":dbl, "y":dbl}[])
                    n287 = Delete From Array(array=w997, length=1, index=0) -> (array with subset deleted=w996:cluster{"x":dbl, "y":dbl}[])  [unwired: 1 out]
                    n288 = local write "Speed"(w996) -> ()
                  }
                }
              }
            }
            n289 = local read "Status"() -> (w977:string)
          }
          frame "CS" {
            w1000 = T2."Enabled" ("Disabled")
            n290 = local write "Connection Lamp"(TRUE) -> ()
            n291 = local write "connection status"("You have successfully connected controller") -> ()
            n292 = property on="X+ 2" class="Bool"("DisabledEnum"=w1000) -> ()  [unwired: 2 in, 2 out]
            n293 = property on="X- 2" class="Bool"("DisabledEnum"=w1000) -> ()  [unwired: 2 in, 2 out]
            n294 = property on="Set Origin" class="Bool"("DisabledEnum"=w1000) -> ()  [unwired: 2 in, 2 out]
            n295 = property on="Back to Home Button 2" class="Bool"("DisabledEnum"=w1000) -> ()  [unwired: 2 in, 2 out]
            n296 = property on="Z- 2" class="Bool"("DisabledEnum"=w1000) -> ()  [unwired: 2 in, 2 out]
            n297 = property on="Y+ 2" class="Bool"("DisabledEnum"=w1000) -> ()  [unwired: 2 in, 2 out]
            n298 = property on="Z+ 2" class="Bool"("DisabledEnum"=w1000) -> ()  [unwired: 2 in, 2 out]
            n299 = property on="Y- 2" class="Bool"("DisabledEnum"=w1000) -> ()  [unwired: 2 in, 2 out]
            n300 = property on="Spindle OFF" class="Bool"("DisabledEnum"=w1000) -> ()  [unwired: 2 in, 2 out]
            n301 = property on="Execute" class="Bool"("DisabledEnum"=w1000) -> ()  [unwired: 2 in, 2 out]
            n302 = property on="set feed rate" class="Bool"("DisabledEnum"=w1000) -> ()  [unwired: 2 in, 2 out]
            n303 = property on="Stop" class="Bool"("DisabledEnum"=w1000) -> ()  [unwired: 2 in, 2 out]
            n304 = property on="Transfer" class="Bool"("DisabledEnum"=w1000) -> ()  [unwired: 2 in, 2 out]
            n305 = property on="set spindle speed" class="Bool"("DisabledEnum"=w1000) -> ()  [unwired: 2 in, 2 out]
            n306 = property on="Clear Graph" class="Bool (strict)"("DisabledEnum"=w1000) -> ()  [unwired: 2 in, 2 out]
            n307 = property on="Spindle ON" class="Bool"("DisabledEnum"=w1000) -> ()  [unwired: 2 in, 2 out]
            n308 = property on="Direction" class="Bool (strict)"("DisabledEnum"=w1000) -> ()  [unwired: 2 in, 2 out]
            n309 = property on="Spindle Speed Knob" class="Knob (strict)"("DisabledEnum"=w1000) -> ()  [unwired: 2 in, 2 out]
            n310 = property on="Feed Rate Knob" class="Knob (strict)"("DisabledEnum"=w1000) -> ()  [unwired: 2 in, 2 out]
            n311 = property on="Spindle Speed" class="DigNum (strict)"("DisabledEnum"=w1000) -> ()  [unwired: 2 in, 2 out]
            n312 = property on="Feed Rate" class="DigNum (strict)"("DisabledEnum"=w1000) -> ()  [unwired: 2 in, 2 out]
            n313 = property on="Address" class="Path"("DisabledEnum"=w1000) -> ()  [unwired: 2 in, 2 out]
            n314 = property on="Save" class="Bool (strict)"("DisabledEnum"=w1000) -> ()  [unwired: 2 in, 2 out]
            n315 = property on="Back to Origin" class="Bool"("DisabledEnum"=w1000) -> ()  [unwired: 2 in, 2 out]
            n316 = property on="Insert" class="Bool (strict)"("DisabledEnum"=w1000) -> ()  [unwired: 2 in, 2 out]
            n317 = property on="Length per Step" class="CmbBox"("DisabledEnum"=w1000) -> ()  [unwired: 2 in, 2 out]
            n318 = property on="Clear" class="Bool (strict)"("DisabledEnum"=w1000) -> ()  [unwired: 2 in, 2 out]
          }
          frame "EMG" {
            w1004 = T2."Disabled and Grayed Out" ("Disabled")
            n319 = local write "Yellow"(FALSE) -> ()
            n320 = local write "Green"(FALSE) -> ()
            n321 = local write "Red"(TRUE) -> ()
            n322 = local read "Status"() -> (w1010:string)
            n323 = Equal?(x=w1010, y="") -> (x = y?=w1009:bool)
            n324 = case shown="False" w1009 {
              tunnel: "Emergency condition, release the button\nthen reset the program for the next use" -> [w1014 w1017]
              tunnel: [w1013 w1017] -> w1008
              frame False {
                n325 = local read "Status"() -> (w1016:string)
                n326 = Concatenate Strings(w1016, "\r", w1014) -> (w1013:string)
              }
              frame True {
              }
            }
            n327 = property on="X+ 2" class="Bool"("DisabledEnum"=w1004) -> ()  [unwired: 2 in, 2 out]
            n328 = property on="X- 2" class="Bool"("DisabledEnum"=w1004) -> ()  [unwired: 2 in, 2 out]
            n329 = property on="Set Origin" class="Bool"("DisabledEnum"=w1004) -> ()  [unwired: 2 in, 2 out]
            n330 = property on="Back to Home Button 2" class="Bool"("DisabledEnum"=w1004) -> ()  [unwired: 2 in, 2 out]
            n331 = property on="Z- 2" class="Bool"("DisabledEnum"=w1004) -> ()  [unwired: 2 in, 2 out]
            n332 = property on="Y+ 2" class="Bool"("DisabledEnum"=w1004) -> ()  [unwired: 2 in, 2 out]
            n333 = property on="Z+ 2" class="Bool"("DisabledEnum"=w1004) -> ()  [unwired: 2 in, 2 out]
            n334 = property on="Y- 2" class="Bool"("DisabledEnum"=w1004) -> ()  [unwired: 2 in, 2 out]
            n335 = property on="Spindle OFF" class="Bool"("DisabledEnum"=w1004) -> ()  [unwired: 2 in, 2 out]
            n336 = property on="Execute" class="Bool"("DisabledEnum"=w1004) -> ()  [unwired: 2 in, 2 out]
            n337 = property on="set feed rate" class="Bool"("DisabledEnum"=w1004) -> ()  [unwired: 2 in, 2 out]
            n338 = property on="Stop" class="Bool"("DisabledEnum"=w1004) -> ()  [unwired: 2 in, 2 out]
            n339 = property on="Transfer" class="Bool"("DisabledEnum"=w1004) -> ()  [unwired: 2 in, 2 out]
            n340 = property on="set spindle speed" class="Bool"("DisabledEnum"=w1004) -> ()  [unwired: 2 in, 2 out]
            n341 = property on="Clear Graph" class="Bool (strict)"("DisabledEnum"=w1004) -> ()  [unwired: 2 in, 2 out]
            n342 = property on="Spindle ON" class="Bool"("DisabledEnum"=w1004) -> ()  [unwired: 2 in, 2 out]
            n343 = property on="Direction" class="Bool (strict)"("DisabledEnum"=w1004) -> ()  [unwired: 2 in, 2 out]
            n344 = property on="Spindle Speed Knob" class="Knob (strict)"("DisabledEnum"=w1004) -> ()  [unwired: 2 in, 2 out]
            n345 = property on="Feed Rate Knob" class="Knob (strict)"("DisabledEnum"=w1004) -> ()  [unwired: 2 in, 2 out]
            n346 = property on="Spindle Speed" class="DigNum (strict)"("DisabledEnum"=w1004) -> ()  [unwired: 2 in, 2 out]
            n347 = property on="Feed Rate" class="DigNum (strict)"("DisabledEnum"=w1004) -> ()  [unwired: 2 in, 2 out]
            n348 = property on="Address" class="Path"("DisabledEnum"=w1004) -> ()  [unwired: 2 in, 2 out]
            n349 = property on="Save" class="Bool (strict)"("DisabledEnum"=w1004) -> ()  [unwired: 2 in, 2 out]
            n350 = property on="Back to Origin" class="Bool"("DisabledEnum"=w1004) -> ()  [unwired: 2 in, 2 out]
            n351 = property on="Insert" class="Bool (strict)"("DisabledEnum"=w1004) -> ()  [unwired: 2 in, 2 out]
            n352 = property on="Length per Step" class="CmbBox"("DisabledEnum"=w1004) -> ()  [unwired: 2 in, 2 out]
            n353 = property on="Clear" class="Bool (strict)"("DisabledEnum"=w1004) -> ()  [unwired: 2 in, 2 out]
          }
          frame "RST" {
            w1018 = T2."Enabled" ("Disabled")
            w1022 = FALSE
            w1020 = 0.0
            w1019 = ""
            n354 = local write "Yellow"(TRUE) -> ()
            n355 = local write "Green"(FALSE) -> ()
            n356 = local write "Red"(FALSE) -> ()
            n357 = local read "Status"() -> (w1028:string)
            n358 = local write "Connection Lamp"(w1022) -> ()
            n359 = local write "Connect Button"(w1022) -> ()
            n360 = local write "Data Receive"(w1019) -> ()
            n361 = local write "Length per Step"(w1019) -> ()
            n362 = local write "G-Code List"(w1019) -> ()
            n363 = local write "Dir"(w1019) -> ()
            n364 = local write "Address"(path " " ("FILE ADDRESS")) -> ()
            n365 = local write "X"(w1020) -> ()
            n366 = local write "Y"(w1020) -> ()
            n367 = local write "Z"(w1020) -> ()
            n368 = local write "Feed Rate"(w1020) -> ()
            n369 = local write "Spindle Speed"(w1020) -> ()
            n370 = local write "Feed Rate Knob"(w1020) -> ()
            n371 = local write "Kp"(w1020) -> ()
            n372 = local write "Kd"(w1020) -> ()
            n373 = local write "Ki"(w1020) -> ()
            n374 = Equal?(x=w1028, y="") -> (x = y?=w1027:bool)
            n375 = case shown="False" w1027 {
              tunnel: "Machine is ready to use" -> [w1032 w1035]
              tunnel: [w1031 w1035] -> w1026
              frame False {
                n376 = local read "Status"() -> (w1034:string)
                n377 = Concatenate Strings(w1034, "\r", w1032) -> (w1031:string)
              }
              frame True {
              }
            }
            n378 = property on="X+ 2" class="Bool"("DisabledEnum"=w1018) -> ()  [unwired: 2 in, 2 out]
            n379 = property on="X- 2" class="Bool"("DisabledEnum"=w1018) -> ()  [unwired: 2 in, 2 out]
            n380 = property on="Set Origin" class="Bool"("DisabledEnum"=w1018) -> ()  [unwired: 2 in, 2 out]
            n381 = property on="Back to Home Button 2" class="Bool"("DisabledEnum"=w1018) -> ()  [unwired: 2 in, 2 out]
            n382 = property on="Z- 2" class="Bool"("DisabledEnum"=w1018) -> ()  [unwired: 2 in, 2 out]
            n383 = property on="Y+ 2" class="Bool"("DisabledEnum"=w1018) -> ()  [unwired: 2 in, 2 out]
            n384 = property on="Z+ 2" class="Bool"("DisabledEnum"=w1018) -> ()  [unwired: 2 in, 2 out]
            n385 = property on="Y- 2" class="Bool"("DisabledEnum"=w1018) -> ()  [unwired: 2 in, 2 out]
            n386 = property on="Spindle OFF" class="Bool"("DisabledEnum"=w1018) -> ()  [unwired: 2 in, 2 out]
            n387 = property on="Execute" class="Bool"("DisabledEnum"=w1018) -> ()  [unwired: 2 in, 2 out]
            n388 = property on="set feed rate" class="Bool"("DisabledEnum"=w1018) -> ()  [unwired: 2 in, 2 out]
            n389 = property on="Stop" class="Bool"("DisabledEnum"=w1018) -> ()  [unwired: 2 in, 2 out]
            n390 = property on="Transfer" class="Bool"("DisabledEnum"=w1018) -> ()  [unwired: 2 in, 2 out]
            n391 = property on="set spindle speed" class="Bool"("DisabledEnum"=w1018) -> ()  [unwired: 2 in, 2 out]
            n392 = property on="Clear Graph" class="Bool (strict)"("DisabledEnum"=w1018) -> ()  [unwired: 2 in, 2 out]
            n393 = property on="Spindle ON" class="Bool"("DisabledEnum"=w1018) -> ()  [unwired: 2 in, 2 out]
            n394 = property on="Direction" class="Bool (strict)"("DisabledEnum"=w1018) -> ()  [unwired: 2 in, 2 out]
            n395 = property on="Spindle Speed Knob" class="Knob (strict)"("DisabledEnum"=w1018) -> ()  [unwired: 2 in, 2 out]
            n396 = property on="Feed Rate Knob" class="Knob (strict)"("DisabledEnum"=w1018) -> ()  [unwired: 2 in, 2 out]
            n397 = property on="Spindle Speed" class="DigNum (strict)"("DisabledEnum"=w1018) -> ()  [unwired: 2 in, 2 out]
            n398 = property on="Feed Rate" class="DigNum (strict)"("DisabledEnum"=w1018) -> ()  [unwired: 2 in, 2 out]
            n399 = property on="Address" class="Path"("DisabledEnum"=w1018) -> ()  [unwired: 2 in, 2 out]
            n400 = property on="Save" class="Bool (strict)"("DisabledEnum"=w1018) -> ()  [unwired: 2 in, 2 out]
            n401 = property on="Back to Origin" class="Bool"("DisabledEnum"=w1018) -> ()  [unwired: 2 in, 2 out]
            n402 = property on="Insert" class="Bool (strict)"("DisabledEnum"=w1018) -> ()  [unwired: 2 in, 2 out]
            n403 = property on="Length per Step" class="CmbBox"("DisabledEnum"=w1018) -> ()  [unwired: 2 in, 2 out]
            n404 = property on="Clear" class="Bool (strict)"("DisabledEnum"=w1018) -> ()  [unwired: 2 in, 2 out]
          }
          frame "HP" {
            n405 = local read "Status"() -> (w1038:string)
            n406 = Equal?(x=w1038, y="") -> (x = y?=w1037:bool)
            n407 = case shown="False" w1037 {
              tunnel: "Arrived in home position" -> [w1042 w1045]
              tunnel: [w1041 w1045] -> w1036
              frame False {
                n408 = local read "Status"() -> (w1044:string)
                n409 = Concatenate Strings(w1044, "\r", w1042) -> (w1041:string)
              }
              frame True {
              }
            }
          }
          frame "ORI" {
            n410 = local read "Status"() -> (w1048:string)
            n411 = Equal?(x=w1048, y="") -> (x = y?=w1047:bool)
            n412 = case shown="False" w1047 {
              tunnel: "Arrived in origin position" -> [w1052 w1055]
              tunnel: [w1051 w1055] -> w1046
              frame False {
                n413 = local read "Status"() -> (w1054:string)
                n414 = Concatenate Strings(w1054, "\r", w1052) -> (w1051:string)
              }
              frame True {
              }
            }
          }
          frame "DC" {
            n415 = local write "Connection Lamp"(FALSE) -> ()
            n416 = local read "Status"() -> (w1059:string)
            n417 = Equal?(x=w1059, y="") -> (x = y?=w1058:bool)
            n418 = case shown="False" w1058 {
              tunnel: "You have disconnected to controller" -> [w1063 w1066]
              tunnel: [w1062 w1066] -> w1057
              frame False {
                n419 = local read "Status"() -> (w1065:string)
                n420 = Concatenate Strings(w1065, "\r", w1063) -> (w1062:string)
              }
              frame True {
              }
            }
          }
          frame "STOP" {
            n421 = local read "Status"() -> (w1069:string)
            n422 = Equal?(x=w1069, y="") -> (x = y?=w1068:bool)
            n423 = case shown="False" w1068 {
              tunnel: "The program is on hold. You may continue the process,\nclick execute." -> [w1073 w1076]
              tunnel: [w1072 w1076] -> w1067
              frame False {
                n424 = local read "Status"() -> (w1075:string)
                n425 = Concatenate Strings(w1075, "\r", w1073) -> (w1072:string)
              }
              frame True {
              }
            }
          }
        }
        n426 = property on="Status" class="Str"("Text.Scroll Position"=w898) -> ()  [unwired: 2 in, 2 out]
        n427 = local write "Status"(w894) -> ()
      }
      n428 = while {
        tunnel: w75 -> [w691]
        tunnel: w74 -> [w690]
        tunnel: [w689] -> w73
        i -> [w685]
        stop <- w689 stop-if-true
        # "524288"
        # "262144"
        # "131072"
        # "65536"
        # "32768"
        # "8192"
        # "4096"
        # "2048"
        # "1024"
        # "512"
        # "16384"
        # "256"
        # "128"
        # "64"
        # "32"
        # "16"
        # "8"
        # "4"
        # "2"
        # "1"
        # "Send Loop"
        n429 = Build Array("X+ 2", "X- 2", "Y+ 2", "Y- 2", "Z+ 2", "Z- 2", "Back to Home Button 2", "Set Origin", "Back to Origin", "Stop", "Spindle ON", "Spindle OFF", "Execute", "Emergency", "Transfer", "Reset", "set feed rate", "set spindle speed", "Feeed Rate Default", "Spindle Speed Default") -> (w694:bool[])
        n430 = Boolean Array To Number(Boolean array=w694) -> (number=w695:u32)
        n431 = case shown="262144" w695 {
          tunnel: w691 -> [w697 w702 w722 w742 w762 w781 w801 w821 w826 w830 w834 w839 w854 w858 w862 w865 w870 w876 w883 w887 w891]
          tunnel: w690 -> [w698 w701 w721 w741 w761 w782 w802 w822 w825 w829 w832 w837 w851 w856 w860 w864 w868 w877 w884 w886 w889]
          tunnel: [w696 w700 w720 w740 w760 w780 w800 w820 w824 w828 w833 w838 w853 w857 w861 w863 w869 w875 w882 w885 w890] -> w689
          tunnel: "Direction" -> [_ _ _ _ _ _ _ _ _ _ _ w836 _ _ _ _ _ _ _ _ _]
          frame 0, Default {
            n432 = TCP Write(connection ID=w698, data in="", error in (no error)=w697) -> (error out=w696:errorcluster)  [unwired: 1 in, 2 out]
          }
          frame 1 {
            n433 = local read "Length per Step"() -> (w703:string)
            n434 = case shown="\"1 mm\"" w703 {
              tunnel: w702 -> [w705 w709 w713 w718]
              tunnel: w701 -> [w706 w710 w714 w716]
              tunnel: [w704 w708 w712 w717] -> w700
              frame "0.1 mm", Default {
                n435 = TCP Write(connection ID=w706, data in="x+0.1", error in (no error)=w705) -> (error out=w704:errorcluster)  [unwired: 1 in, 2 out]
              }
              frame "1 mm" {
                n436 = TCP Write(connection ID=w710, data in="x+1", error in (no error)=w709) -> (error out=w708:errorcluster)  [unwired: 1 in, 2 out]
              }
              frame "10 mm" {
                n437 = TCP Write(connection ID=w714, data in="x+10", error in (no error)=w713) -> (error out=w712:errorcluster)  [unwired: 1 in, 2 out]
              }
              frame "100 mm" {
                n438 = TCP Write(connection ID=w716, data in="x+100", error in (no error)=w718) -> (error out=w717:errorcluster)  [unwired: 1 in, 2 out]
              }
            }
          }
          frame 2 {
            n439 = local read "Length per Step"() -> (w723:string)
            n440 = case shown="\"0.1 mm\", Default" w723 {
              tunnel: w722 -> [w726 w731 w734 w738]
              tunnel: w721 -> [w725 w730 w733 w737]
              tunnel: [w724 w729 w732 w736] -> w720
              frame "0.1 mm", Default {
                n441 = TCP Write(connection ID=w725, data in="x-0.1", error in (no error)=w726) -> (error out=w724:errorcluster)  [unwired: 1 in, 2 out]
              }
              frame "1 mm" {
                n442 = TCP Write(connection ID=w730, data in="x-1", error in (no error)=w731) -> (error out=w729:errorcluster)  [unwired: 1 in, 2 out]
              }
              frame "10 mm" {
                n443 = TCP Write(connection ID=w733, data in="x-10", error in (no error)=w734) -> (error out=w732:errorcluster)  [unwired: 1 in, 2 out]
              }
              frame "100 mm" {
                n444 = TCP Write(connection ID=w737, data in="x-100", error in (no error)=w738) -> (error out=w736:errorcluster)  [unwired: 1 in, 2 out]
              }
            }
          }
          frame 4 {
            n445 = local read "Length per Step"() -> (w743:string)
            n446 = case shown="\"1 mm\"" w743 {
              tunnel: w742 -> [w746 w750 w754 w757]
              tunnel: w741 -> [w745 w748 w752 w756]
              tunnel: [w744 w749 w753 w758] -> w740
              frame "0.1 mm", Default {
                n447 = TCP Write(connection ID=w745, data in="y+0.1", error in (no error)=w746) -> (error out=w744:errorcluster)  [unwired: 1 in, 2 out]
              }
              frame "1 mm" {
                n448 = TCP Write(connection ID=w748, data in="y+1", error in (no error)=w750) -> (error out=w749:errorcluster)  [unwired: 1 in, 2 out]
              }
              frame "10 mm" {
                n449 = TCP Write(connection ID=w752, data in="y+10", error in (no error)=w754) -> (error out=w753:errorcluster)  [unwired: 1 in, 2 out]
              }
              frame "100 mm" {
                n450 = TCP Write(connection ID=w756, data in="y+100", error in (no error)=w757) -> (error out=w758:errorcluster)  [unwired: 1 in, 2 out]
              }
            }
          }
          frame 8 {
            n451 = local read "Length per Step"() -> (w763:string)
            n452 = case shown="\"0.1 mm\", Default" w763 {
              tunnel: w762 -> [w766 w770 w774 w778]
              tunnel: w761 -> [w765 w769 w773 w777]
              tunnel: [w764 w768 w772 w776] -> w760
              frame "0.1 mm", Default {
                n453 = TCP Write(connection ID=w765, data in="y-0.1", error in (no error)=w766) -> (error out=w764:errorcluster)  [unwired: 1 in, 2 out]
              }
              frame "1 mm" {
                n454 = TCP Write(connection ID=w769, data in="y-1", error in (no error)=w770) -> (error out=w768:errorcluster)  [unwired: 1 in, 2 out]
              }
              frame "10 mm" {
                n455 = TCP Write(connection ID=w773, data in="y-10", error in (no error)=w774) -> (error out=w772:errorcluster)  [unwired: 1 in, 2 out]
              }
              frame "100 mm" {
                n456 = TCP Write(connection ID=w777, data in="y-100", error in (no error)=w778) -> (error out=w776:errorcluster)  [unwired: 1 in, 2 out]
              }
            }
          }
          frame 16 {
            n457 = local read "Length per Step"() -> (w783:string)
            n458 = case shown="\"1 mm\"" w783 {
              tunnel: w782 -> [w785 w789 w793 w797]
              tunnel: w781 -> [w786 w790 w794 w798]
              tunnel: [w784 w788 w792 w796] -> w780
              frame "0.1 mm", Default {
                n459 = TCP Write(connection ID=w785, data in="z+0.1", error in (no error)=w786) -> (error out=w784:errorcluster)  [unwired: 1 in, 2 out]
              }
              frame "1 mm" {
                n460 = TCP Write(connection ID=w789, data in="z+1", error in (no error)=w790) -> (error out=w788:errorcluster)  [unwired: 1 in, 2 out]
              }
              frame "10 mm" {
                n461 = TCP Write(connection ID=w793, data in="z+10", error in (no error)=w794) -> (error out=w792:errorcluster)  [unwired: 1 in, 2 out]
              }
              frame "100 mm" {
                n462 = TCP Write(connection ID=w797, data in="z+100", error in (no error)=w798) -> (error out=w796:errorcluster)  [unwired: 1 in, 2 out]
              }
            }
          }
          frame 32 {
            n463 = local read "Length per Step"() -> (w803:string)
            n464 = case shown="\"1 mm\"" w803 {
              tunnel: w802 -> [w806 w808 w814 w818]
              tunnel: w801 -> [w805 w810 w813 w817]
              tunnel: [w804 w809 w812 w816] -> w800
              frame "0.1 mm", Default {
                n465 = TCP Write(connection ID=w806, data in="z-0.1", error in (no error)=w805) -> (error out=w804:errorcluster)  [unwired: 1 in, 2 out]
              }
              frame "1 mm" {
                n466 = TCP Write(connection ID=w808, data in="z-1", error in (no error)=w810) -> (error out=w809:errorcluster)  [unwired: 1 in, 2 out]
              }
              frame "10 mm" {
                n467 = TCP Write(connection ID=w814, data in="z-10", error in (no error)=w813) -> (error out=w812:errorcluster)  [unwired: 1 in, 2 out]
              }
              frame "100 mm" {
                n468 = TCP Write(connection ID=w818, data in="z-100", error in (no error)=w817) -> (error out=w816:errorcluster)  [unwired: 1 in, 2 out]
              }
            }
          }
          frame 64 {
            n469 = TCP Write(connection ID=w822, data in="home", error in (no error)=w821) -> (error out=w820:errorcluster)  [unwired: 1 in, 2 out]
          }
          frame 128 {
            n470 = TCP Write(connection ID=w825, data in="set0", error in (no error)=w826) -> (error out=w824:errorcluster)  [unwired: 1 in, 2 out]
          }
          frame 256 {
            n471 = TCP Write(connection ID=w829, data in="ori", error in (no error)=w830) -> (error out=w828:errorcluster)  [unwired: 1 in, 2 out]
          }
          frame 512 {
            n472 = TCP Write(connection ID=w832, data in="stop", error in (no error)=w834) -> (error out=w833:errorcluster)  [unwired: 1 in, 2 out]
          }
          frame 1024 {
            n473 = case shown="False" w836 {
              tunnel: w839 -> [w843 w848]
              tunnel: [w842 w847] -> w838
              tunnel: w837 -> [w841 w846]
              frame False {
                n474 = TCP Write(connection ID=w841, data in="cw", error in (no error)=w843) -> (error out=w842:errorcluster)  [unwired: 1 in, 2 out]
                n475 = local write "Dir"("cw") -> ()
              }
              frame True {
                n476 = TCP Write(connection ID=w846, data in="ccw", error in (no error)=w848) -> (error out=w847:errorcluster)  [unwired: 1 in, 2 out]
                n477 = local write "Dir"("ccw") -> ()
              }
            }
          }
          frame 2048 {
            n478 = local write "Spindle Lamp"(FALSE) -> ()
            n479 = TCP Write(connection ID=w851, data in="spin0", error in (no error)=w854) -> (error out=w853:errorcluster)  [unwired: 1 in, 2 out]
          }
          frame 4096 {
            n480 = TCP Write(connection ID=w856, data in="start", error in (no error)=w858) -> (error out=w857:errorcluster)  [unwired: 1 in, 2 out]
          }
          frame 8192 {
            n481 = TCP Write(connection ID=w860, data in="emg", error in (no error)=w862) -> (error out=w861:errorcluster)  [unwired: 1 in, 2 out]
          }
          frame 16384 {
            n482 = local read "G-Code List"() -> (w866:string)
            n483 = TCP Write(connection ID=w864, data in=w866, error in (no error)=w865) -> (error out=w863:errorcluster)  [unwired: 1 in, 2 out]
          }
          frame 32768 {
            n484 = TCP Write(connection ID=w868, data in="rst", error in (no error)=w870) -> (error out=w869:errorcluster)  [unwired: 1 in, 2 out]
          }
          frame 65536 {
            n485 = local read "Feed Rate"() -> (w874:dbl)
            n486 = Number To Decimal String(number=w874) -> (decimal integer string=w872:string)  [unwired: 1 in]
            n487 = Concatenate Strings("f", w872) -> (w871:string)
            n488 = TCP Write(connection ID=w877, data in=w871, error in (no error)=w876) -> (error out=w875:errorcluster)  [unwired: 1 in, 2 out]
          }
          frame 131072 {
            n489 = local read "Spindle Speed"() -> (w881:dbl)
            n490 = Number To Decimal String(number=w881) -> (decimal integer string=w879:string)  [unwired: 1 in]
            n491 = Concatenate Strings("s", w879) -> (w878:string)
            n492 = TCP Write(connection ID=w884, data in=w878, error in (no error)=w883) -> (error out=w882:errorcluster)  [unwired: 1 in, 2 out]
          }
          frame 262144 {
            n493 = TCP Write(connection ID=w886, data in="df", error in (no error)=w887) -> (error out=w885:errorcluster)  [unwired: 1 in, 2 out]
          }
          frame 524288 {
            n494 = TCP Write(connection ID=w889, data in="ds", error in (no error)=w891) -> (error out=w890:errorcluster)  [unwired: 1 in, 2 out]
          }
        }
        n495 = property on="Status" class="Str"("Text.Scroll Position"=w685) -> ()  [unwired: 2 in, 2 out]
      }
      n496 = Merge Errors(w76, w73) -> (w72:errorcluster)
    }
    frame Error {
      n497 = local write "Connection Lamp"(FALSE) -> ()
      n498 = local write "connection status"("Connection failed. Input a correct IP address!") -> ()
    }
  }
  n499 = while {
    stop <- FALSE stop-if-true
    n500 = event shown="[2] \"About\": Mouse Up" {
      selector: _ -> [_ _ _]
      dyn-events: _ -> [_ _ _]
      timeout: _ -> [_ _ _]
      event "Help": Mouse Up {
        n501 = event-data() -> ()  [unwired: 1 in, 8 out]
        n502 = case shown="True" "Help" {
          frame False {
          }
          frame True {
            n503 = One Button Dialog(message="HELP\nThis program is used to control a CNC Engraving Machine\n", button name ("OK")="OK" ("message")) -> ()  [unwired: 1 out]
          }
        }
      }
      event "Exit Program": Mouse Up {
        n504 = event-data() -> ()  [unwired: 1 in, 8 out]
        n505 = case shown="True" "Exit Program" {
          frame False {
          }
          frame True {
            n506 = Two Button Dialog(message="Are you sure want to close the program?", 1:"No" ("F button name (\"Cancel\")"), 2:"Yes" ("T button name (\"OK\")")) -> (T button?=w1086:bool)
            n507 = case shown="True" w1086 {
              frame False {
              }
              frame True {
                n508 = local read "Connection Lamp"() -> (w1090:bool)
                n509 = case shown="True" w1090 {
                  selector: w1090 -> [w1092 _]
                  frame False {
                    n510 = Not(x=w1092) -> (.not. x?=w1091:bool)
                    n511 = Quit LabVIEW(quit? (T)=w1091) -> ()
                  }
                  frame True {
                    n512 = One Button Dialog(message="Connection with machine still detected!\nPlease stop all current process and disconnect the controller before exiting the program!") -> ()  [unwired: 1 in, 1 out]
                  }
                }
              }
            }
          }
        }
      }
      event "About": Mouse Up {
        n513 = event-data() -> ()  [unwired: 1 in, 8 out]
        n514 = case shown="True" "About" {
          frame False {
          }
          frame True {
            n515 = One Button Dialog(message="ABOUT\n3D CNC Engraving using Raspberry Controller with TCP/IP Data Communication by C1 2019.\n1. Muhamad Pribadi Lukman (216341061)\n2. Muhammad Edo Fadilah (216341062)\n3. Fitri Wineka (216341058)\n4. Aisyah Nur Afiati (216341050)  ", button name ("OK")="OK" ("message")) -> ()  [unwired: 1 out]
          }
        }
      }
    }
  }
  n516 = TCP Close Connection(connection ID=w4, error in (no error)=w6) -> (error out=w5:errorcluster)  [unwired: 1 in, 1 out]
  n517 = call <vilib>:"Simple Error Handler.vi"("error in (no error)"=w5) -> ()  [unwired: 4 in, 5 out]
